vi "main.vi"() -> ()   [LabVIEW 2025]
uses:
  Controls/States.ctl
  Controls/HR_Data_Structure.ctl
  Controls/Raw_Data_IN_HR.ctl
  Controls/Runner_Data_Structure.ctl
  <vilib>/Analysis/baseanly.llb/Mean (DBL).vi
  <vilib>/Analysis/NI_AALBase.lvlib
panel:
  out "FATIGUE":cluster{"Time":timestamp[], "Array":dbl[]}(graph)
  out "BPM":cluster{"Time":timestamp[], "Bpm":i32[]}(graph)
  out "Zone PLOT":T1(graph)
  out "Zone Data":string[][](array[string]) caption="HEART RATE ZONES"
  in  "File Path":path
  out "error out":errorcluster
  in  "error in":errorcluster
  in  "Stop":bool
  in  "Save Results":bool
  in  "New Training":bool
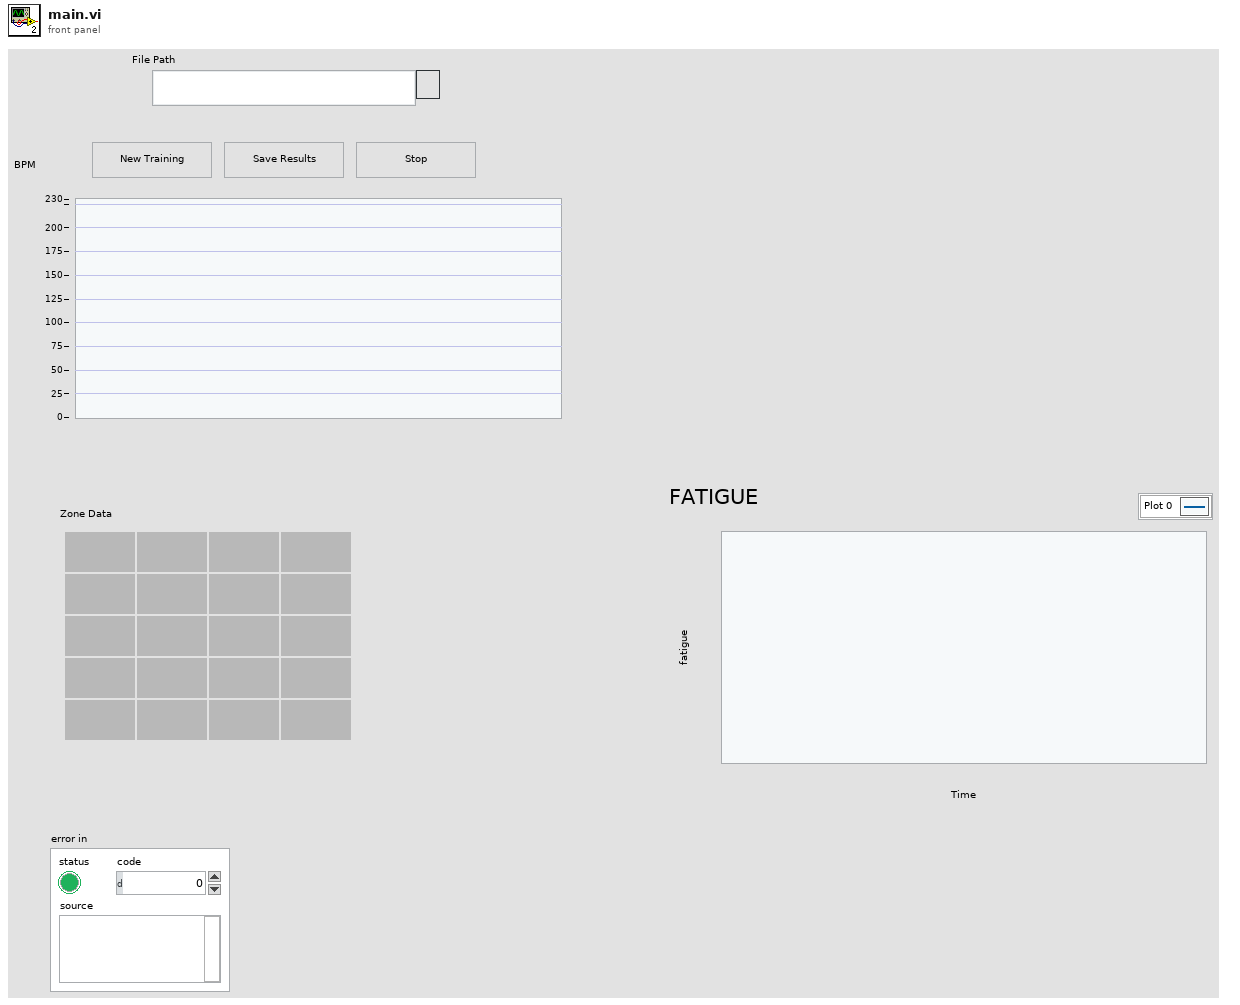
[diagram p1: front panel]
types:
  T1 = cluster{"Total Time in Zone":dbl[], "Heart Rate Zone No":dbl[]}
  T2 = typedef "HR_Data_Structure.ctl" = cluster{"HR Max":i32, "% HR MAX ":dbl[], "Raw Data":T3, "Runner's Data":T4, "HR Zone":string[][], "Total Time in Zone":dbl[], "Heart Rate Zone No":dbl[]}
  T3 = typedef "Raw_Data_IN_HR.ctl" = cluster{"Time":timestamp[], "Bpm":i32[]}
  T4 = typedef "Runner_Data_Structure.ctl" = cluster{"Name":string, "Age":i32}
  T5 = typedef "States.ctl" = enum16{"Application Error", "Init", "Idle", "Analyse New Training", "Save", "Error Handling", "Stop"}
  T6 = enum16{"open", "replace", "create", "open or create", "replace or create", "replace or create with confirmation"}
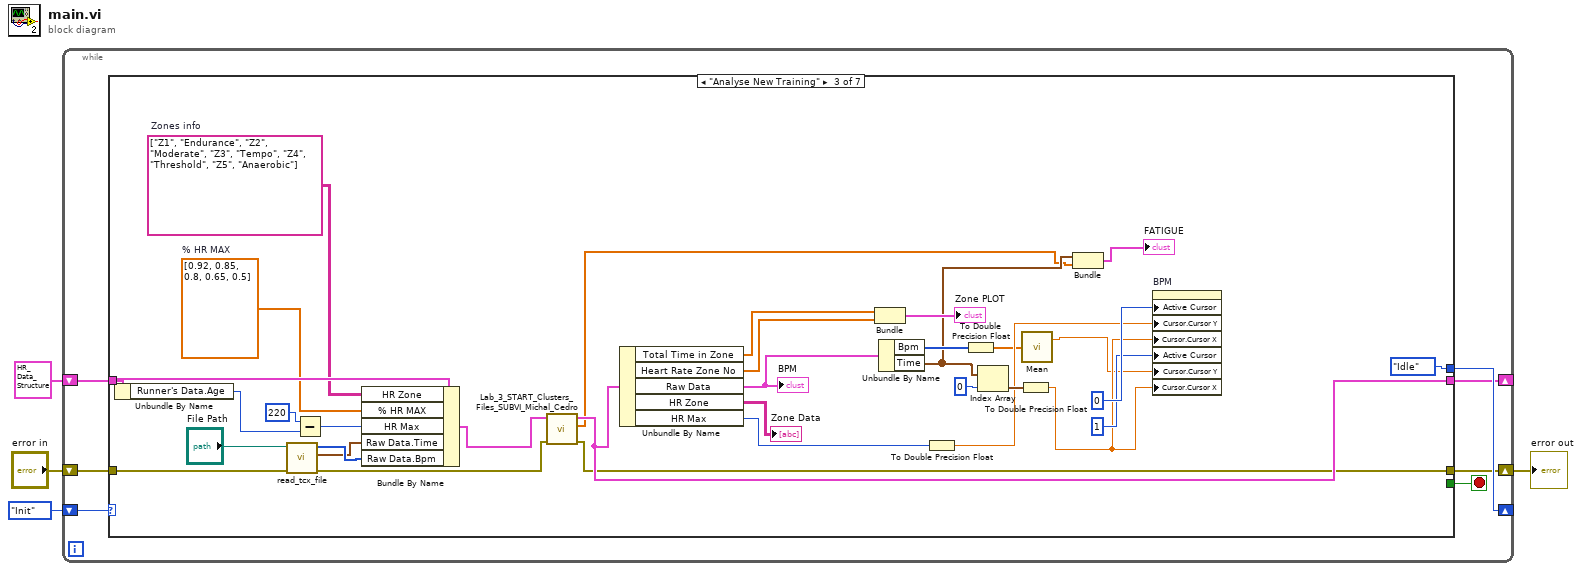
[diagram p0: block diagram]
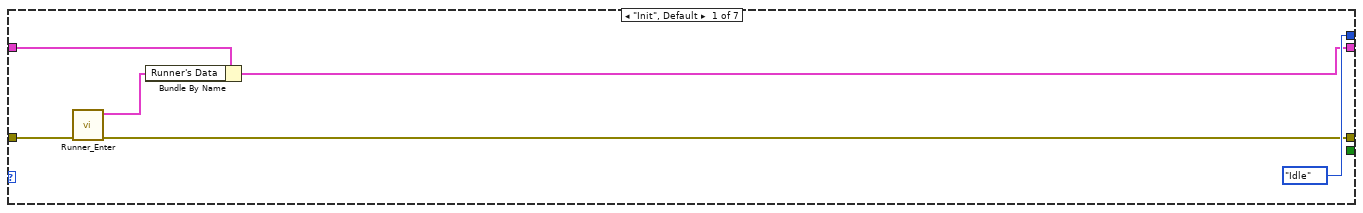
[diagram p2: hidden frame]
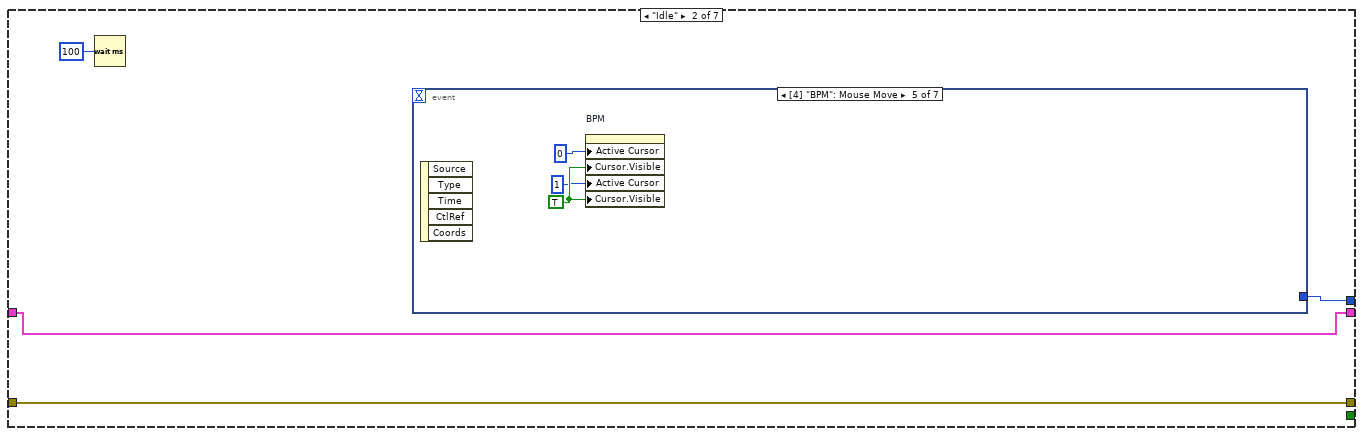
[diagram p3: hidden frame]
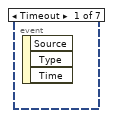
[diagram p4: hidden frame]
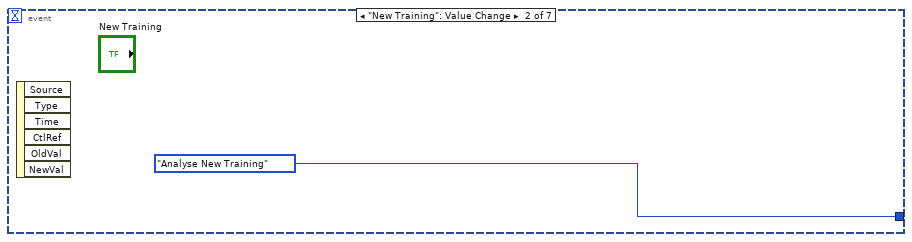
[diagram p5: hidden frame]
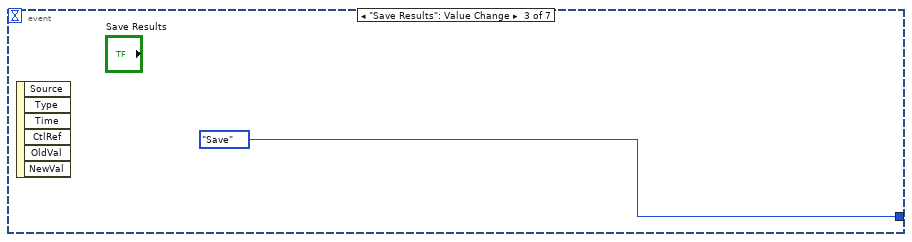
[diagram p6: hidden frame]
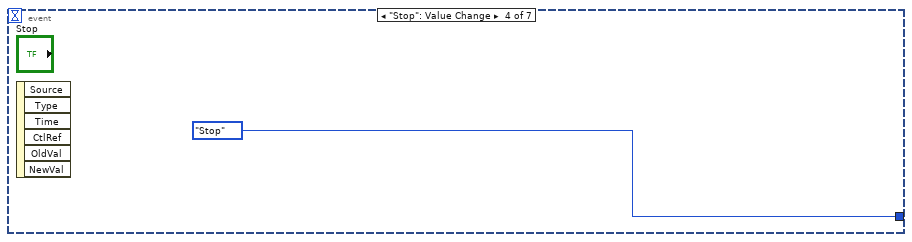
[diagram p7: hidden frame]
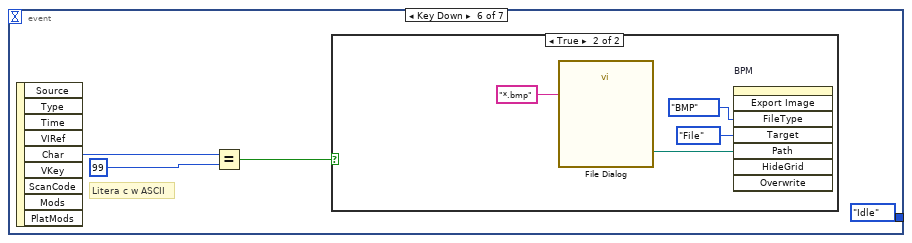
[diagram p8: hidden frame]
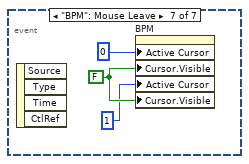
[diagram p10: hidden frame]
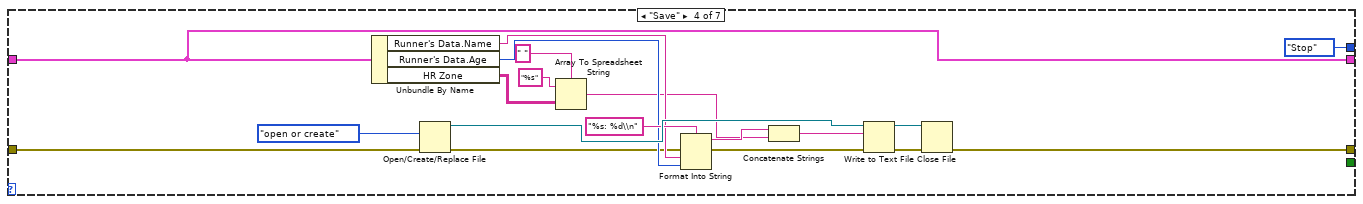
[diagram p11: hidden frame]
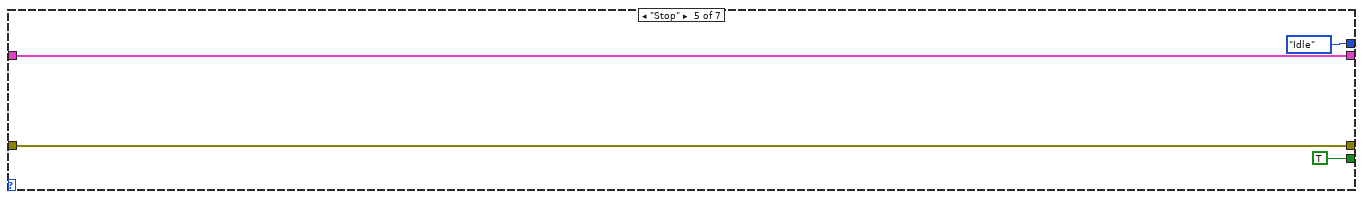
[diagram p12: hidden frame]
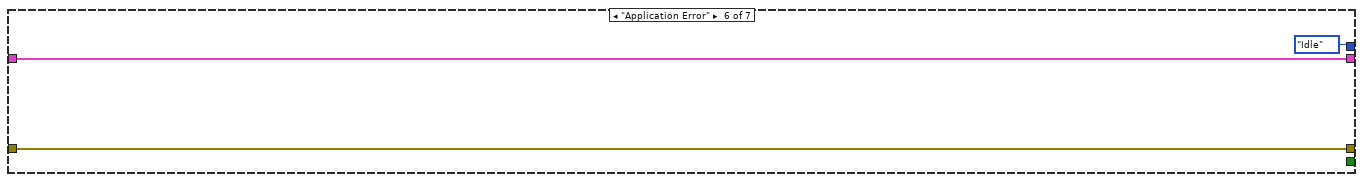
[diagram p13: hidden frame]
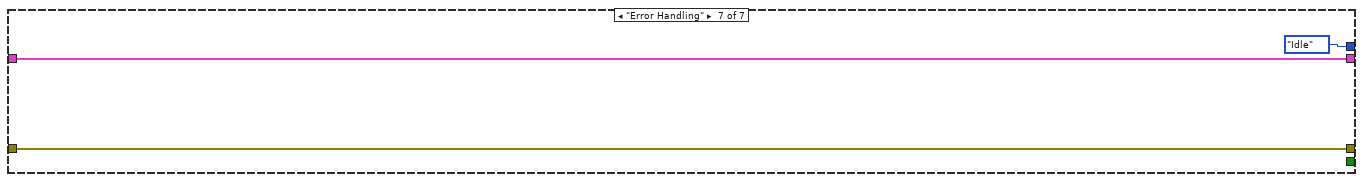
[diagram p14: hidden frame]
diagram:
  n1 = while {
    shift-right: [w11] -> _
    shift-left: States."Init" -> [w5]
    shift-right: [w8] -> _
    shift-left: T2 data[18004B] ("HR Data Structure 2") -> [w7]
    shift-right: [w9] -> w2
    shift-left: "error in" -> [w10]
    stop <- w6 stop-if-true
    n2 = case shown="\"Analyse New Training\"" w5 {
      tunnel: [States."Idle" w19 States."Idle" States."Stop" States."Idle" States."Idle" States."Idle"] -> w11
      tunnel: w10 -> [w15 w21 w65 w88 w93 w95 w99]
      tunnel: [w14 w21 w42 w85 w93 w95 w99] -> w9
      tunnel: [w13 w18 w45 w84 w92 w96 w100] -> w8
      tunnel: w7 -> [w12 w18 w62 w84 w92 w96 w100]
      tunnel: [_ _ _ _ TRUE _ _] -> w6
      frame "Init", Default {
        n3 = call "Runner_Enter.vi"("error in"=w15) -> ("error out"=w14:errorcluster, "Runner's Data OUT"=w17:T4)  [unwired: 9 in]
        n4 = Bundle By Name(cluster=w12, "Runner's Data"=w17) -> (w13:T2)
      }
      frame "Idle" {
        n5 = Wait (ms)(milliseconds to wait=u32 100) -> ()  [unwired: 1 out]
        n6 = event shown="[4] \"BPM\": Mouse Move" {
          selector: _ -> [_ _ _ _ _ _ _]
          dyn-events: _ -> [_ _ _ _ _ _ _]
          timeout: _ -> [_ _ _ _ _ _ _]
          tunnel: [_ States."Analyse New Training" States."Save" States."Stop" _ States."Idle" _] -> w19
          event Timeout {
            n7 = event-data() -> ()  [unwired: 1 in, 3 out]
          }
          event "New Training": Value Change {
            n8 = event-data() -> ()  [unwired: 1 in, 6 out]
          }
          event "Save Results": Value Change {
            n9 = event-data() -> ()  [unwired: 1 in, 6 out]
          }
          event "Stop": Value Change {
            n10 = event-data() -> ()  [unwired: 1 in, 6 out]
          }
          event "BPM": Mouse Move {
            w27 = TRUE
            n11 = event-data() -> ()  [unwired: 1 in, 5 out]
            n12 = property on="BPM" class="XYGraph (strict)"("Active Cursor"=u32 0, "Cursor.Visible"=w27, "Active Cursor"=u32 1, "Cursor.Visible"=w27) -> ()  [unwired: 2 in, 2 out]
          }
          event Key Down {
            # "Litera c w ASCII"
            n13 = event-data() -> ("Char"=w31:i16)  [unwired: 1 in, 8 out]
            n14 = Equal?(x=w31, y=i16 99) -> (x = y?=w28:bool)
            n15 = case shown="True" w28 {
              frame False {
              }
              frame True {
                n16 = call "File Dialog"("pattern (all files)"="*.bmp" ("pattern label")) -> ("selected path"=w33:path)  [unwired: 11 in, 3 out]
                n17 = invoke on="BPM" class="XYGraph (strict)" method="Export Image"("FileType"=enum32{"BMP", "EPS", "EMF", "PICT"}."BMP" ("File Type"), "Target"=enum32{"File", "Clipboard"}."File", "Path"=w33) -> ()  [unwired: 5 in, 8 out]
              }
            }
          }
          event "BPM": Mouse Leave {
            w38 = FALSE
            n18 = event-data() -> ()  [unwired: 1 in, 4 out]
            n19 = property on="BPM" class="XYGraph (strict)"("Active Cursor"=u32 0, "Cursor.Visible"=w38, "Active Cursor"=u32 1, "Cursor.Visible"=w38) -> ()  [unwired: 2 in, 2 out]
          }
        }
      }
      frame "Analyse New Training" {
        w44 = string[][] [["Z1", "Endurance"], ["Z2", "Moderate"], ["Z3", "Tempo"], ["Z4", "Threshold"], ["Z5", "Anaerobic"]]  # Zones info
        w43 = dbl[] [0.92, 0.85, 0.8, 0.65, 0.5]  # % HR MAX
        n20 = Unbundle By Name(w62) -> ("Runner's Data.Age"=w71:i32)
        n21 = call "read_tcx_file.vi"("error in"=w65, "File Path"="File Path") -> ("error out"=w47:errorcluster, "Time"=w57:timestamp[], "Bpm"=w64:i32[])  [unwired: 7 in]
        n22 = Subtract(x=220, y=w71) -> (x-y=w60:i32)
        n23 = Bundle By Name(cluster=w62, "HR Zone"=w44, "% HR MAX"=w43, "HR Max"=w60, "Raw Data.Time"=w57, "Raw Data.Bpm"=w64) -> (w46:T2)
        n24 = call "Lab_3_START_Clusters_Files_SUBVI_Michal_Cedro.vi"("Error IN"=w47, "HR Data Structure IN"=w46) -> ("error out"=w42:errorcluster, "Array"=w39:dbl[], "HR Data Structure OUT"=w45:T2)  [unwired: 7 in]
        n25 = Unbundle By Name(w45) -> ("Total Time in Zone"=w66:dbl[], "Heart Rate Zone No"=w67:dbl[], "Raw Data"=w49:T3, "HR Zone"=→"Zone Data":string[][], "HR Max"=w53:i32)
        "BPM" <- w49
        n26 = Bundle("Total Time in Zone"=w66, "Heart Rate Zone No"=w67) -> (→"Zone PLOT":T1)  [unwired: 1 in]
        n27 = Unbundle By Name(w49) -> ("Bpm"=w50:i32[], "Time"=w40:timestamp[])
        n28 = To Double Precision Float(number=w53) -> (double precision float=w52:dbl)
        n29 = To Double Precision Float(number=w50) -> (double precision float=w51:dbl[])
        n30 = Index Array(array=w40, index=0) -> (element=w55:timestamp)
        n31 = To Double Precision Float(number=w55) -> (double precision float=w54:dbl)
        n32 = call-poly <vilib>:"Mean.vi"("X"=w51) -> ("mean"=w48:dbl)  [unwired: 1 out]
        n33 = Bundle("Time"=w40, "Array"=w39) -> (→"FATIGUE":cluster{"Time":timestamp[], "Array":dbl[]})  [unwired: 1 in]
        n34 = property on="BPM" class="XYGraph (strict)"("Active Cursor"=u32 0, "Cursor.Cursor Y"=w52, "Cursor.Cursor X"=w54, "Active Cursor"=u32 1, "Cursor.Cursor Y"=w48, "Cursor.Cursor X"=w54) -> ()  [unwired: 2 in, 2 out]
      }
      frame "Save" {
        n35 = Unbundle By Name(w84) -> ("Runner's Data.Name"=w82:string, "Runner's Data.Age"=w81:i32, "HR Zone"=w78:string[][])
        n36 = Open/Create/Replace File(error in=w88, operation (0:open)=T6."open or create") -> (refnum out=w89:refnum<file>, error out=w80:errorcluster)  [unwired: 4 in, 1 out]
        n37 = Array To Spreadsheet String(delimiter (Tab)=" ", array=w78, 3:"%s" ("format string")) -> (spreadsheet string=w76:string)
        n38 = Format Into String(format string="%s: %d\\n", error in=w80, w82, w81) -> (resulting string=w77:string, error out=w79:errorcluster)  [unwired: 1 in]
        n39 = Concatenate Strings(w77, w76) -> (w75:string)
        n40 = Write to Text File(file (use dialog)=w89, text=w75, error in=w79) -> (refnum out=w87:refnum<file>, error out=w86:errorcluster)  [unwired: 1 in, 1 out]
        n41 = Close File(refnum=w87, error in=w86) -> (error out=w85:errorcluster)  [unwired: 1 out]
      }
      frame "Stop" {
      }
      frame "Application Error" {
      }
      frame "Error Handling" {
      }
    }
  }
  "error out" <- w2
